vi "CheckForOnlineDevices.vi"(8 "error in (no error)":errorcluster, 11 "service":refnum<class "IcmMessageService.lvclass">) -> (0 "error out":errorcluster)   [LabVIEW 2016]
doc: "Queries for all equipment asset nodes, which means they have operating states."
uses:
  <vilib>/addons/InsightCM/MessageBus/MessageService/IcmMessageService.lvclass
  <vilib>/addons/InsightCM/MessageBus/Base/controls/KeyValuePair.ctl
  <vilib>/addons/InsightCM/MessageBus/Base/controls/MessageHeader.ctl
  <vilib>/addons/InsightCM/MessageBus/MessageLibrary/Device/controls/DevicePingResponse.ctl
panel:
  out "DevicePingResponse":T1
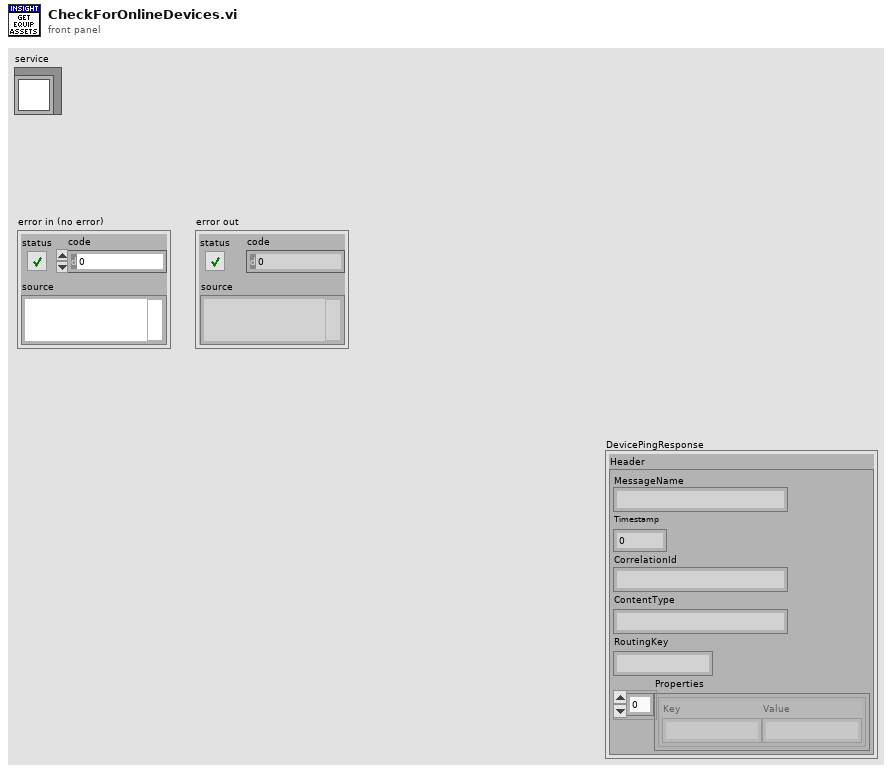
[diagram p1: front panel]
types:
  T1 = typedef "DevicePingResponse.ctl" = cluster{"Header":T2}
  T2 = typedef "MessageHeader.ctl" = cluster{"MessageName":string, "Timestamp":i64, "CorrelationId":string, "ContentType":string, "RoutingKey":string, "Properties":T3[]}
  T3 = typedef "KeyValuePair.ctl" = cluster{"Key":string, "Value":string}
  T4 = typedef "Message.ctl" = cluster{"Header":T2, "Body":u8[]}
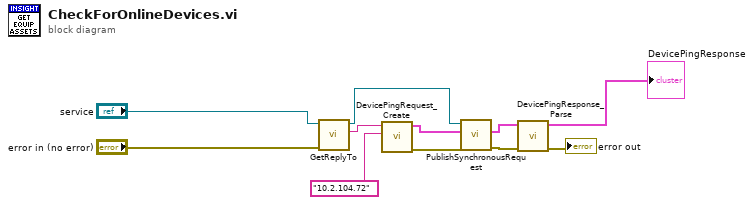
[diagram p0: block diagram]
diagram:
  n1 = call <vilib>:"GetReplyTo.vi"("error in (no error)"="error in (no error)", "service in"="service") -> ("reply to"=w8:string, "service out"=w9:refnum<class "IcmMessageService.lvclass">)  [unwired: 7 in, 1 out]
  n2 = call <vilib>:"DevicePingRequest_Create.vi"("SendTo"="10.2.104.72", "ReplyTo"=w8) -> ("error out"=w7:errorcluster, "Message"=w6:T4)  [unwired: 8 in]
  n3 = call <vilib>:"PublishSynchronousRequest.vi"("error in (no error)"=w7, "request"=w6, "service in"=w9) -> ("error out"=w5:errorcluster, "response"=w4:T4)  [unwired: 6 in, 1 out]
  n4 = call <vilib>:"DevicePingResponse_Parse.vi"("error in (no error)"=w5, "Message"=w4) -> ("error out"=→"error out":errorcluster, "DevicePingResponse"=→"DevicePingResponse":T1)  [unwired: 7 in, 1 out]
